vi "Read processing parameters.vi"(8 "error in (no error)":errorcluster, 11 "Shared Memory Runtime in":refnum<class "Shared Memory Runtime.lvclass">) -> (0 "error out":errorcluster, 2 "processing parameters":T1[](array[typedef]), 3 "Shared Memory Runtime out":refnum<class "Shared Memory Runtime.lvclass">)   [LabVIEW 2013, in "Shared Memory Runtime.lvclass"]
uses:
  Shared Memory Runtime.lvclass
  shared memory module runtime.ctl
  <vilib>/NI/Tag Bus Module Framework/channel/channel classification.ctl
  <vilib>/NI/Tag Bus/tag/Data Type.ctl
  <vilib>/National Instruments/Shared Memory Library for Linux RT/Controls/Shared Memory Class Reference.ctl
  <vilib>/National Instruments/Shared Memory Library for Linux RT/Classes/Shared Memory/Shared Memory.lvclass
  Shared Memory Runtime.lvclass/Shared Memory Runtime.ctl
  <vilib>/NI/Tag Bus Module Framework/channel/TBM channel.lvclass
  <vilib>/NI/Tag Bus/tag/tag descriptor.lvclass
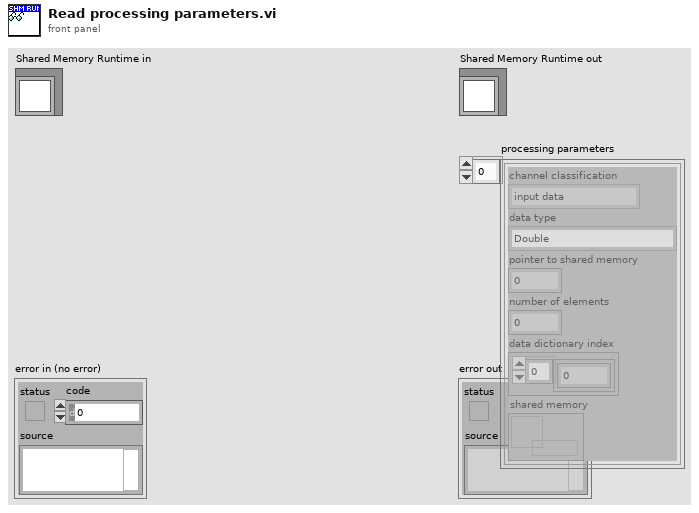
[diagram p1: front panel]
types:
  T1 = typedef "shared memory runtime.lvclass/shared memory module runtime.ctl" = cluster{"channel classification":T2, "data type":T3, "pointer to shared memory":u64, "number of elements":u64, "data dictionary index":cluster{i32[]}, "shared memory":T4}
  T2 = typedef "TBM channel.lvclass/channel classification.ctl" = enum16{"input data", "output data", "processing parameter", "processing result"}
  T3 = typedef "tag bus.lvlib/tag descriptor.lvclass/Data Type.ctl" = enum16{"Double", "Single", "I64", "I32", "I16", "I8", "U64", "U32", "U16", "U8", "Boolean", "String", "Array of Double", "Array of Single", "Array of I64", "Array of I32", "Array of I16", "Array of I8", "Array of U64", "Array of U32", "Array of U16", "Array of U8", "Array of Boolean", "Array of String"}
  T4 = typedef "Shared Memory Class Reference.ctl" = refnum<data-value>
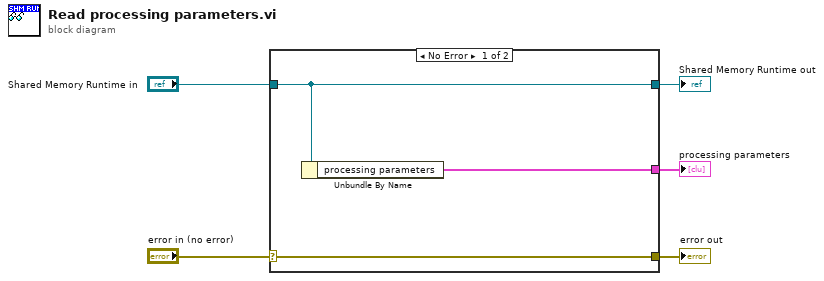
[diagram p0: block diagram]
diagram:
  n1 = case shown="No Error" "error in (no error)" {
    selector: "error in (no error)" -> [w8 w9]
    tunnel: [w8 w9] -> w4
    tunnel: [w7 w10] -> w2
    tunnel: "Shared Memory Runtime in" -> [w7 w10]
    tunnel: [w6 _] -> w1
    frame No Error {
      n2 = Unbundle By Name(w7) -> ("processing parameters"=w6:T1[])
    }
    frame Error {
    }
  }
  "error out" <- w4
  "Shared Memory Runtime out" <- w2
  "processing parameters" <- w1
